vi "SendFLCam_DAC.vi"(0 "ctrl":u8, 1 "feature":u8, 2 "data":u16, 3 "addr":u8) -> ()   [LabVIEW 2015]
uses:
  ESLSCDLL.dll
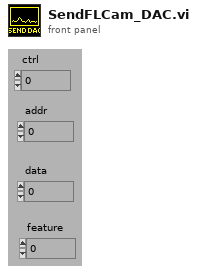
[diagram p1: front panel]
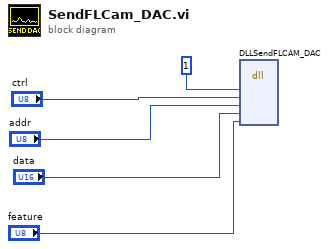
[diagram p0: block diagram]
diagram:
  n1 = dll-call lib="C:/ENTW/PCIE/lv64/lv15_act2018/board.vis/ESLSCDLL.dll" fn="DLLSendFLCAM_DAC" ("lwlscdll.dll:DLLSetADAmpRed")("drvno"=u32 1, "ctrl"="ctrl", "addr"="addr", "data"="data", "feature"="feature") -> ()  [unwired: 9 in, 2 out]
